vi "Run JSL (String).vi"(8 "error in (no error)":errorcluster, 10 "JSL command":string, 11 "JMP application":refnum<k7>) -> (0 "error out":errorcluster, 3 "JMP application out":refnum<k7>)   [LabVIEW 2019, in "JMP Automation.lvlib"]
doc: "Runs JSL text that is provided in string form."
uses:
  JMP Automation.lvlib
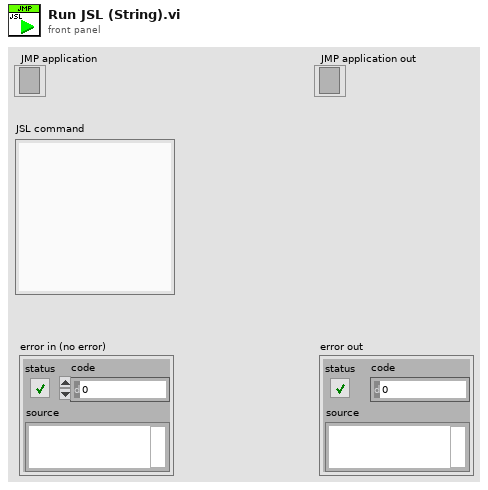
[diagram p1: front panel]
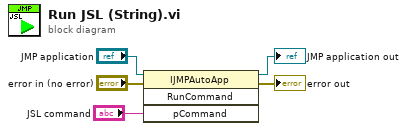
[diagram p0: block diagram]
diagram:
  n1 = invoke class="IJMPAutoApp" method="RunCommand"(reference="JMP application", error in="error in (no error)", "pCommand"="JSL command") -> (reference out=→"JMP application out":refnum<k7>, error out=→"error out":errorcluster)  [unwired: 1 in, 2 out]
